vi "medicaoIXV.vi"() -> ()   [LabVIEW 2012]
uses:
  <vilib>/Utility/file.llb/Write To Spreadsheet File (string).vi
  <vilib>/Utility/file.llb/Write To Spreadsheet File (DBL).vi
  <instrlib>/Agilent 6XXX Series/Agilent 6XXX Series.lvlib
panel:
  out "array":dbl[][](array[numeric])
  in  "Tab Control":enum32{"Entrada de dados", "Saída de dados"}(tab)
  out "ON/OFF":bool
  in  "Pontos":dbl
  in  "Tensão máxima":dbl
  in  "Nome da célula":string
  in  "Local":path
  in  "Delay(ms)":dbl
  in  "Start":bool
  in  "Print Screen":bool
  out "IXV":cluster{"Y":dbl[], "Y":dbl[]}[](graph)
  out "output voltage":dbl
  out "Tensao Atual":dbl
  out "Corrente Atual":dbl
  out "Ponto Atual":i32
  out "TABELA DE DADOS\nTensão(fonte)     Tensão                  Corrente            Pontos":dbl[][](array[numeric]) caption="all rows" format="%0.3f"
  in  "stop":bool
  in  "CorrenteGraph":dbl
  in  "error in (no error)":errorcluster
  out "error out":errorcluster
  in  "TensaoGraph":dbl
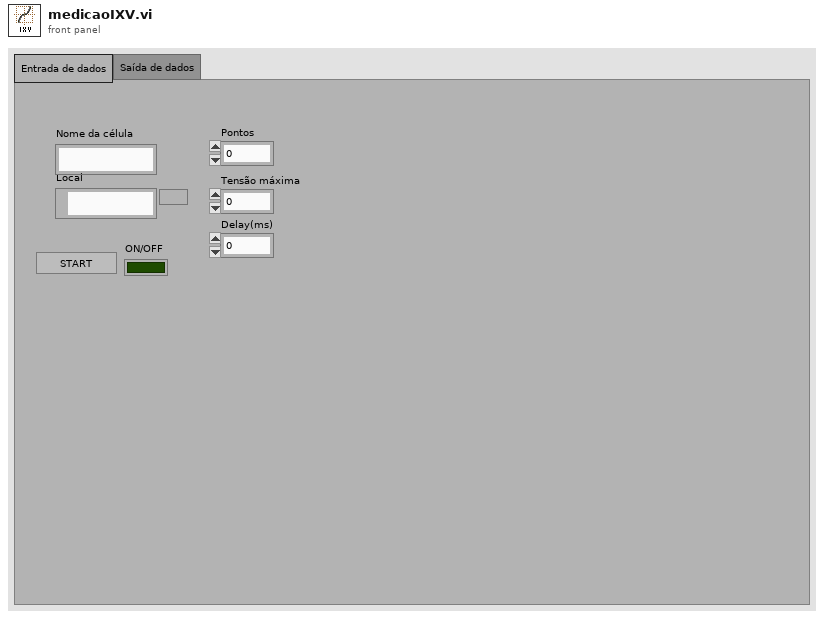
[diagram p1: front panel]
types:
  T1 = typedef "imagedata.ctl" = cluster{"image type":i32, "image depth":i32, "image":u8[], "mask":u8[], "colors":u32[], "Rectangle":cluster{"left":i16, "top":i16, "right":i16, "bottom":i16}}
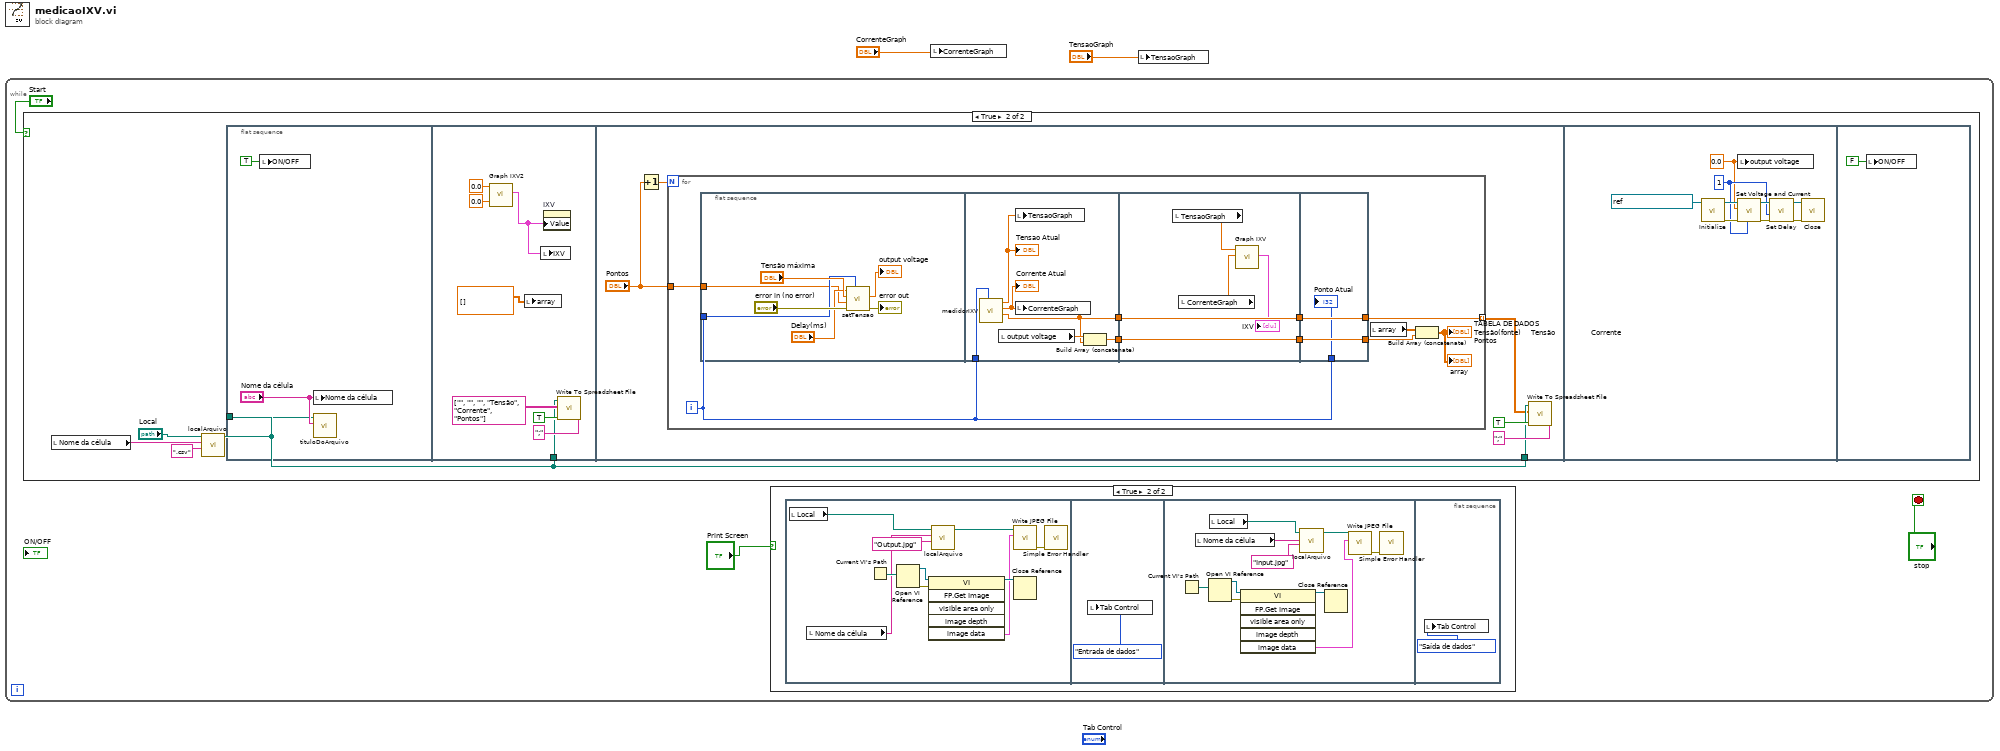
[diagram p0: block diagram]
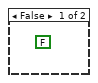
[diagram p3: hidden frame]
diagram:
  n1 = while {
    stop <- "stop" stop-if-true
    n2 = case shown="True" "Start" {
      frame False {
        (unwired) FALSE
      }
      frame True {
        n3 = local read "Nome da célula"() -> (w29:string)
        n4 = call "localArquivo.vi"("extensão"=".csv", "Nome do arquivo"=w29, "Local"="Local") -> ("Path"=w28:path)  [unwired: 8 in]
        n5 = flat-sequence {
          tunnel: w28 -> [w33]
          tunnel: w28 -> [w39]
          tunnel: w28 -> [w46]
          frame #0 {
            n6 = local write "ON/OFF"(TRUE ("ON/OFF")) -> ()
            n7 = local write "Nome da célula"("Nome da célula") -> ()
            n8 = call "tituloDoArquivo.vi"("Nome da célula"="Nome da célula", "file path (dialog if empty)"=w33) -> ()  [unwired: 10 in]
          }
          frame #1 {
            n9 = call "Graph IXV2"("Y Input"=0.0, "X Input"=0.0) -> ("XY Graph"=w35:cluster{"Y":dbl[], "Y":dbl[]}[])  [unwired: 3 in, 6 out]
            n10 = local write "array"(dbl[][] [] ("array")) -> ()
            n11 = local write "IXV"(w35) -> ()
            n12 = property on="IXV" class="XYGraph (strict)"("Value"=w35) -> ()  [unwired: 2 in, 2 out]
            n13 = call-poly <vilib>:"Write To Spreadsheet File.vi"("delimiter (\\t)"=";" ("delimiter (\\t)"), "append to file? (new file:F)"=TRUE, "2D data"=string[][] [["", "", ""], ["Tensão", "Corrente", "Pontos"]], "file path (dialog if empty)"=w39) -> ()  [unwired: 4 in, 1 out]
          }
          frame #2 {
            n14 = Increment(x="Pontos") -> (x+1=w45:dbl)
            n15 = for {
              N: w45 -> [_]
              tunnel: [w57] -> w43 mode=indexing
              tunnel: "Pontos" -> [w58]
              i -> [w49]
              n16 = flat-sequence {
                tunnel: w58 -> [w61]
                tunnel: w49 -> [w62]
                tunnel: w49 -> [w71]
                tunnel: [w66] -> w56
                tunnel: [w68] -> w55
                tunnel: w56 -> [w76]
                tunnel: w55 -> [w75]
                tunnel: [w76] -> w51
                tunnel: [w75] -> w50
                tunnel: [w78] -> w54
                tunnel: [w79] -> w57
                tunnel: w51 -> [w79]
                tunnel: w50 -> [w78]
                tunnel: w49 -> [w77]
                frame #0 {
                  n17 = call "setTensao.vi"("Ponto"=w62, "error in (no error)"="error in (no error)", "Pontos"=w61, "Tensão máxima"="Tensão máxima", "delay(ms)"="Delay(ms)") -> ("error out"=→"error out":errorcluster, "output voltage"=→"output voltage":dbl)  [unwired: 5 in]
                }
                frame #1 {
                  n18 = call "medidorIXV.vi"("Ponto"=w71) -> ("Array"=w66:dbl[], "Corrente Atual"=w70:dbl, "Tensao Atual"=w69:dbl)  [unwired: 8 in]
                  "Corrente Atual" <- w70
                  "Tensao Atual" <- w69
                  n19 = local read "output voltage"() -> (w67:dbl)
                  n20 = local write "TensaoGraph"(w69) -> ()
                  n21 = local write "CorrenteGraph"(w70) -> ()
                  n22 = Build Array (concatenate)(w67, w66) -> (w68:dbl[])
                }
                frame #2 {
                  n23 = local read "TensaoGraph"() -> (w74:dbl)
                  n24 = local read "CorrenteGraph"() -> (w73:dbl)
                  n25 = call "Graph IXV"("Y Input"=w73, "X Input"=w74) -> ("XY Graph"=→"IXV":cluster{"Y":dbl[], "Y":dbl[]}[])  [unwired: 3 in, 6 out]
                }
                frame #3 {
                  "Ponto Atual" <- w77
                }
              }
              n26 = local read "array"() -> (w53:dbl[][])
              n27 = Build Array (concatenate)(w53, w54) -> (→"TABELA DE DADOS\nTensão(fonte)     Tensão                  Corrente            Pontos" →"array":dbl[][])
            }
            n28 = call-poly <vilib>:"Write To Spreadsheet File.vi"("delimiter (\\t)"=";" ("delimiter (\\t)"), "append to file? (new file:F)"=TRUE, "2D data"=w43, "file path (dialog if empty)"=w46) -> ()  [unwired: 4 in, 1 out]
          }
          frame #3 {
            w80 = 0.0 ("voltage (0 V)")
            w83 = u8 1 ("channel (1)")
            n29 = call <instrlib>:"Initialize.vi"("VISA resource name"=refnum<visa-resource-name> "GPIB0::5::INSTR") -> ("error out"=w85:errorcluster, "VISA resource name out"=w84:refnum<visa-resource-name>)  [unwired: 9 in]
            n30 = local write "output voltage"(w80) -> ()
            n31 = call <instrlib>:"Set Voltage and Current.vi"("channel (1)"=w83, "error in (no error)"=w85, "voltage (0 V)"=w80, "VISA resource name"=w84) -> ("error out"=w86:errorcluster, "VISA resource name out"=w87:refnum<visa-resource-name>)  [unwired: 6 in]
            n32 = call <instrlib>:"Set Delay.vi"("error in (no error)"=w86, "channel (1)"=w83, "VISA resource name"=w87) -> ("error out"=w81:errorcluster, "VISA resource name out"=w82:refnum<visa-resource-name>)  [unwired: 7 in]
            n33 = call <instrlib>:"Close.vi"("error in (no error)"=w81, "VISA resource name"=w82) -> ()  [unwired: 9 in, 1 out]
          }
          frame #4 {
            n34 = local write "ON/OFF"(FALSE) -> ()
          }
        }
      }
    }
    n35 = case shown="True" "Print Screen" {
      frame False {
      }
      frame True {
        n36 = flat-sequence {
          frame #0 {
            n37 = local read "Local"() -> (w7:path)
            n38 = local read "Nome da célula"() -> (w6:string)
            n39 = Current VI's Path() -> (path=w12:path)
            n40 = Open VI Reference(vi path=w12) -> (vi reference=w13:refnum<vi>, error out=w14:errorcluster)  [unwired: 5 in]
            n41 = invoke class="VI" method="FP.Get Image"(reference=w13, error in=w14) -> (reference out=w11:refnum<vi>, "image data"=w10:T1)  [unwired: 4 in, 4 out]
            n42 = call "localArquivo.vi"("extensão"="Output.jpg", "Nome do arquivo"=w6, "Local"=w7) -> ("Path"=w15:path)  [unwired: 8 in]
            n43 = call <vilib>:"Write JPEG File.vi"("image data"=w10, "path to JPEG file"=w15) -> ("error out"=w9:errorcluster)  [unwired: 8 in, 1 out]
            n44 = Close Reference(reference=w11) -> ()  [unwired: 1 in, 1 out]
            n45 = call <vilib>:"Simple Error Handler.vi"("error in (no error)"=w9) -> ()  [unwired: 4 in, 5 out]
          }
          frame #1 {
            n46 = local write "Tab Control"(enum32{"Entrada de dados", "Saída de dados"}."Entrada de dados" ("Tab Control")) -> ()
          }
          frame #2 {
            n47 = Current VI's Path() -> (path=w25:path)
            n48 = local read "Nome da célula"() -> (w18:string)
            n49 = Open VI Reference(vi path=w25) -> (vi reference=w24:refnum<vi>, error out=w23:errorcluster)  [unwired: 5 in]
            n50 = local read "Local"() -> (w17:path)
            n51 = invoke class="VI" method="FP.Get Image"(reference=w24, error in=w23) -> (reference out=w26:refnum<vi>, "image data"=w21:T1)  [unwired: 4 in, 4 out]
            n52 = call "localArquivo.vi"("extensão"="Input.jpg", "Nome do arquivo"=w18, "Local"=w17) -> ("Path"=w20:path)  [unwired: 8 in]
            n53 = Close Reference(reference=w26) -> ()  [unwired: 1 in, 1 out]
            n54 = call <vilib>:"Write JPEG File.vi"("image data"=w21, "path to JPEG file"=w20) -> ("error out"=w22:errorcluster)  [unwired: 8 in, 1 out]
            n55 = call <vilib>:"Simple Error Handler.vi"("error in (no error)"=w22) -> ()  [unwired: 4 in, 5 out]
          }
          frame #3 {
            n56 = local write "Tab Control"(enum32{"Entrada de dados", "Saída de dados"}."Saída de dados" ("Tab Control")) -> ()
          }
        }
      }
    }
  }
  n57 = local write "CorrenteGraph"("CorrenteGraph") -> ()
  n58 = local write "TensaoGraph"("TensaoGraph") -> ()
